vi "Vehicle.vi"(8 "error in (no error)":errorcluster, 9 "Logger In":refnum<queue>, 10 "Pipeline In":refnum<queue>, 11 "Vehicle Queue In":refnum<queue>) -> (0 "error out":errorcluster, 3 "Vehicle Queue Out":refnum<queue>)   [LabVIEW 2016]
uses:
  Message Format.ctl
  StateDef_generic.ctl
  StateData_Vehicle.ctl
  <vilib>/addons/zeromq/socket_type.ctl
  <vilib>/addons/zeromq/socket_options.ctl
  <vilib>/addons/zeromq/zmq_socket.lvclass
  <vilib>/addons/zeromq/zmq_context.lvclass
  <vilib>/addons/zeromq/zeromq.lvlib
panel:
  out "Vehicle  Sensors":cluster{dbl, dbl, dbl}(graph)
  # "VEHICLE DATA"
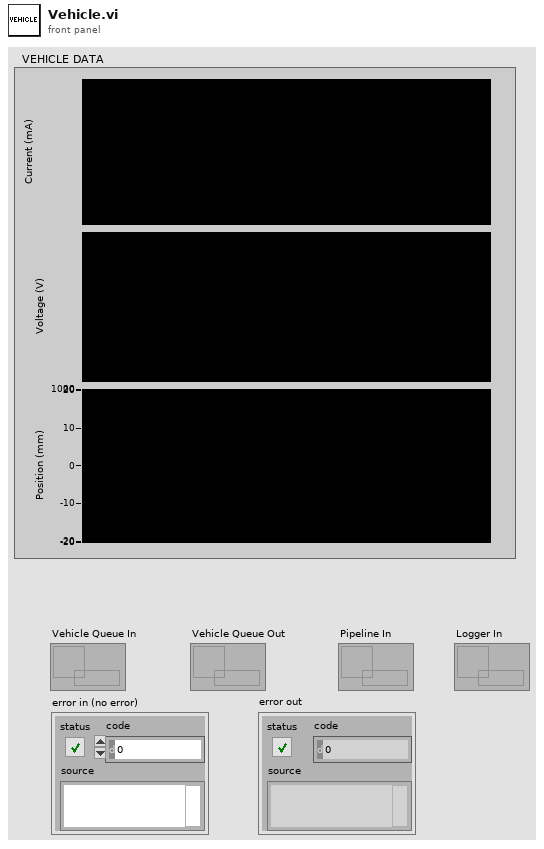
[diagram p1: front panel]
types:
  T1 = typedef "StateData_Vehicle.ctl" = cluster{"Current":dbl, "Voltage":dbl, "Position":dbl}
  T2 = typedef "StateDef_generic.ctl" = enum16{"Initialize", "Running", "Exit"}
  T3 = typedef "zeromq.lvlib/socket_options.ctl" = enum8{"NONE", "ZMQ_HWM", "<2>", "ZMQ_SWAP", "ZMQ_AFFINITY", "ZMQ_IDENTITY", "ZMQ_SUBSCRIBE", "ZMQ_UNSUBSCRIBE", "ZMQ_RATE", "ZMQ_RECOVERY_IVL", "ZMQ_MCAST_LOOP", "ZMQ_SNDBUF", "ZMQ_RCVBUF", "ZMQ_RCVMORE", "ZMQ_FD", "ZMQ_EVENTS", "ZMQ_TYPE", "ZMQ_LINGER", "ZMQ_RECONNECT_IVL", "ZMQ_BACKLOG", "ZMQ_RECOVERY_IVL_MSEC", "ZMQ_RECONNECT_IVL_MAX", "ZMQ_MAXMSGSIZE", "ZMQ_SNDHWM", "ZMQ_RCVHWM", "ZMQ_MULTICAST_HOPS", "<26>", "ZMQ_RCVTIMEO", "ZMQ_SNDTIMEO", "<29>", "<30>", "ZMQ_IPV4ONLY", "ZMQ_LAST_ENDPOINT", "ZMQ_ROUTER_MANDATORY", "ZMQ_TCP_KEEPALIVE", "ZMQ_TCP_KEEPALIVE_CNT", "ZMQ_TCP_KEEPALIVE_IDLE", "ZMQ_TCP_KEEPALIVE_INTVL", "ZMQ_TCP_ACCEPT_FILTER", "ZMQ_DELAY_ATTACH_ON_CONNECT", "ZMQ_XPUB_VERBOSE"}
  T4 = typedef "zeromq.lvlib/socket_type.ctl" = enum8{"ZMQ_PAIR", "ZMQ_PUB", "ZMQ_SUB", "ZMQ_REQ", "ZMQ_REP", "ZMQ_DEALER", "ZMQ_ROUTER", "ZMQ_PULL", "ZMQ_PUSH", "ZMQ_XPUB", "ZMQ_XSUB"}
  T5 = typedef "Message Format.ctl" = cluster{"header":string, "data":variant}
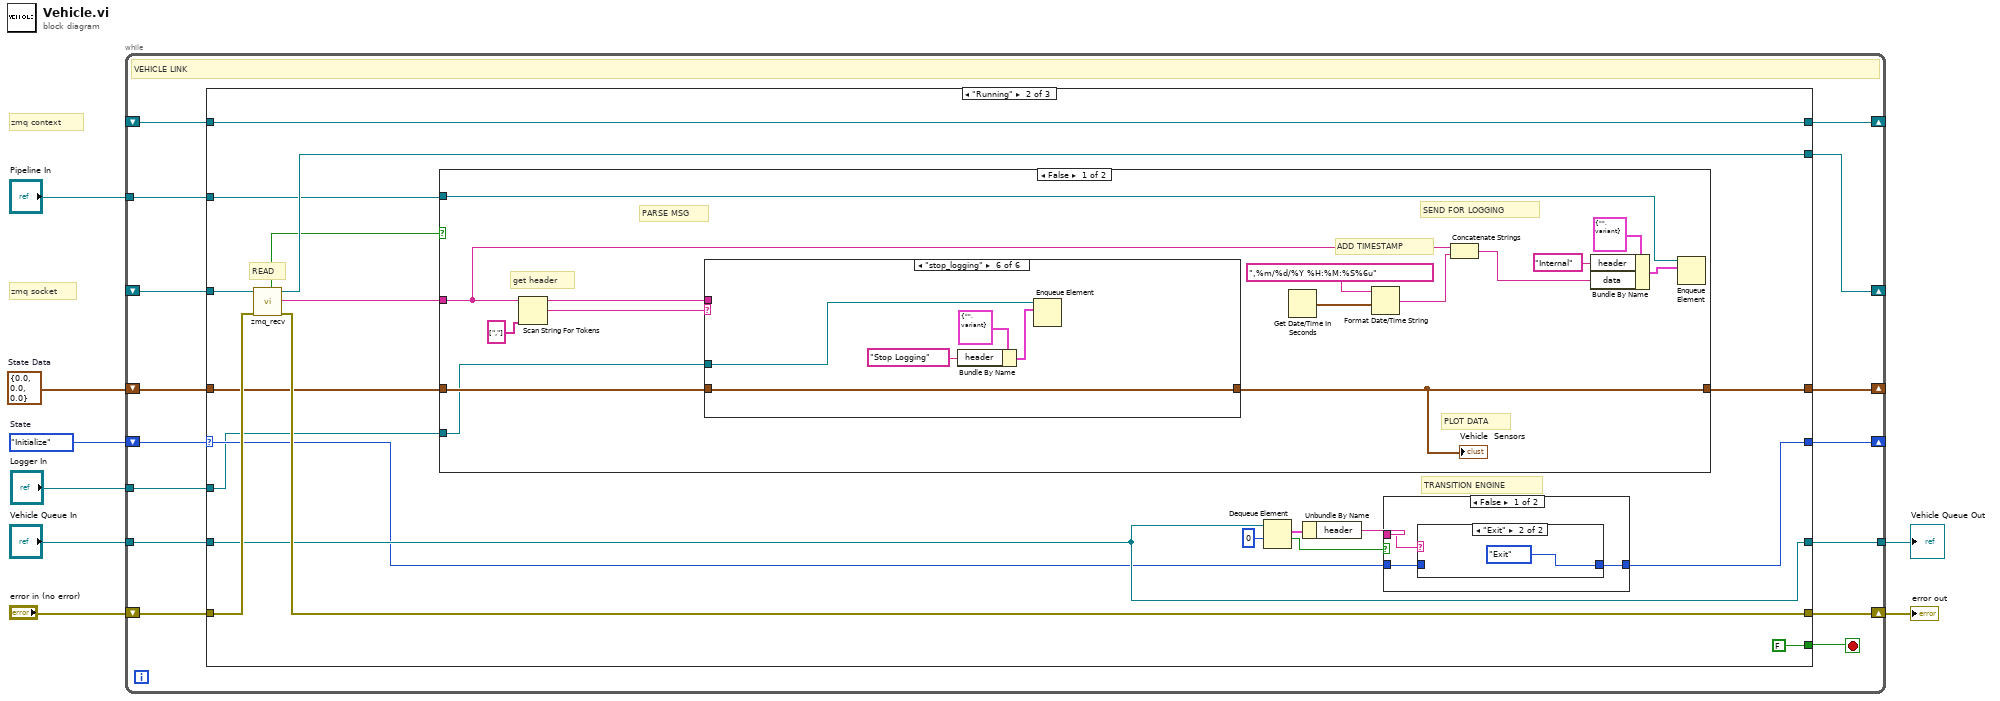
[diagram p0: block diagram]
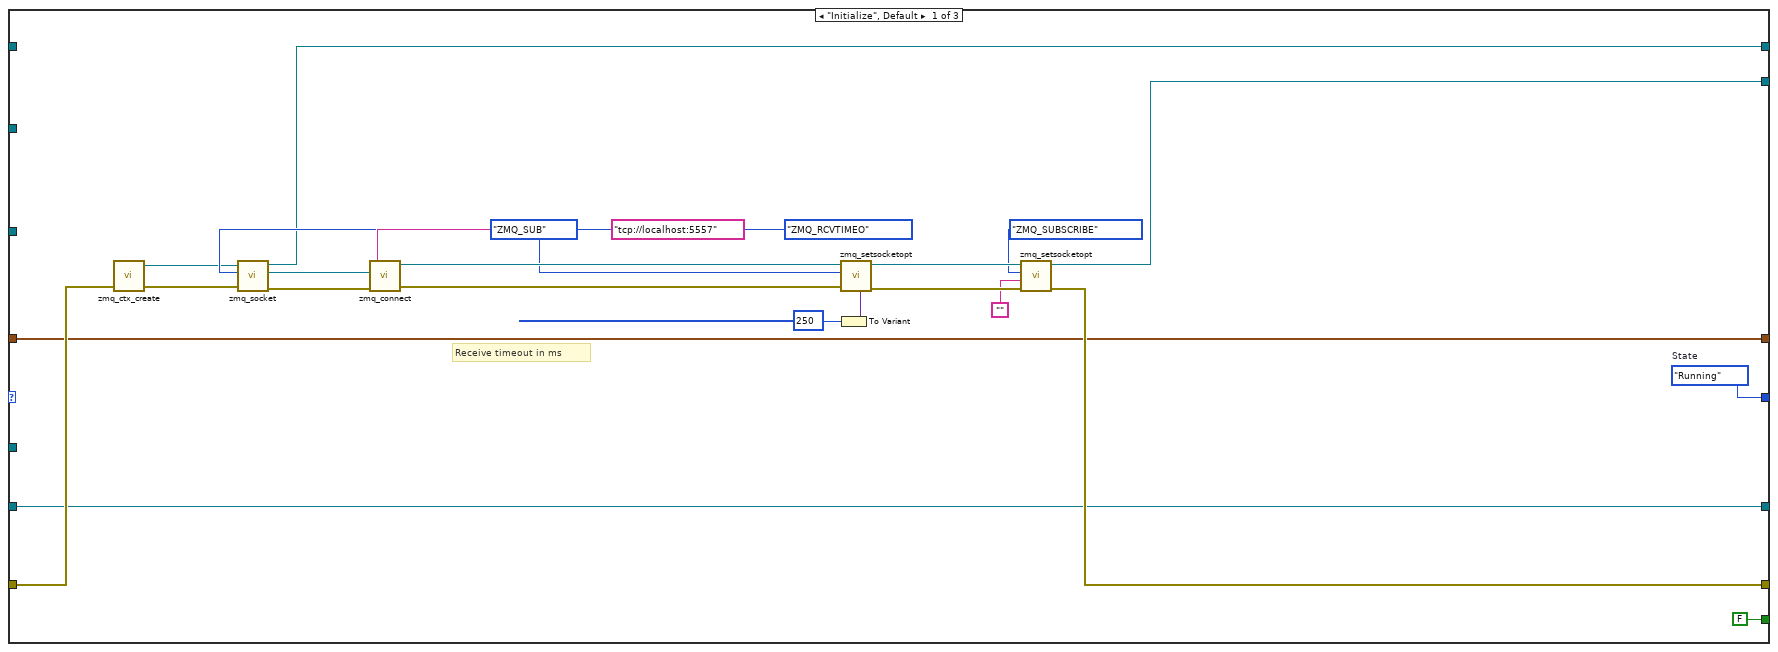
[diagram p2: hidden frame]
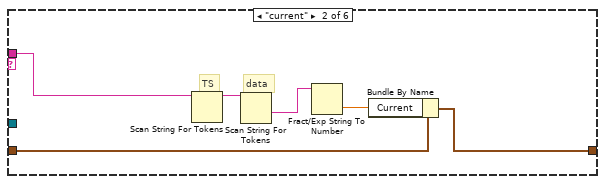
[diagram p6: hidden frame]
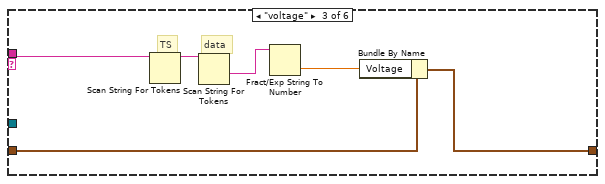
[diagram p7: hidden frame]
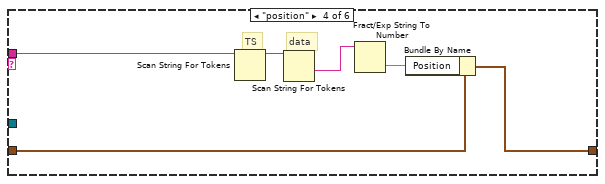
[diagram p8: hidden frame]
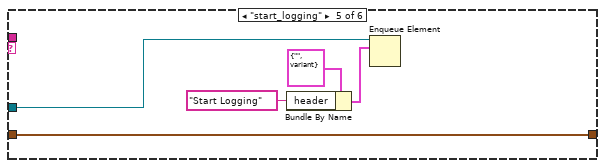
[diagram p9: hidden frame]
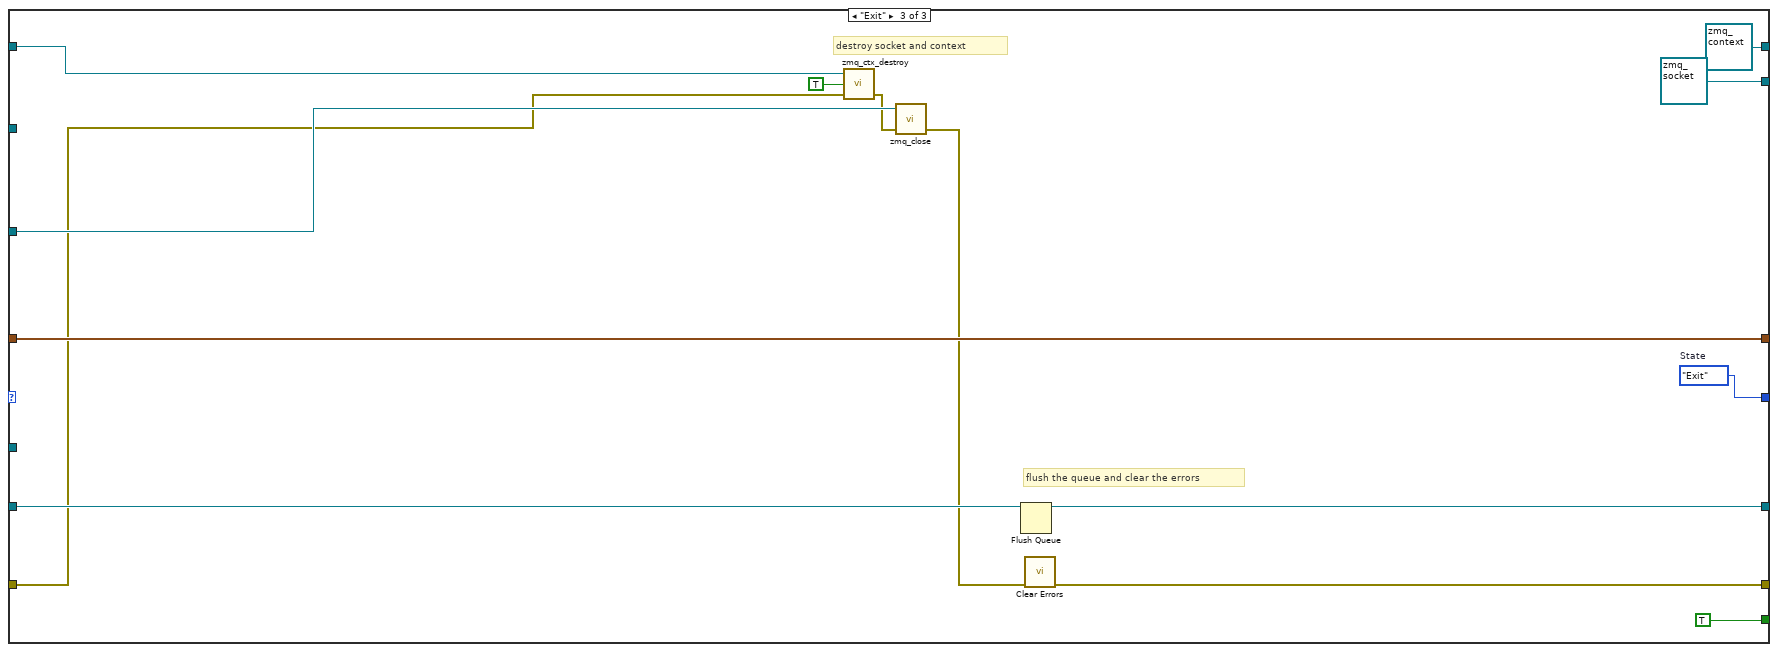
[diagram p11: hidden frame]
diagram:
  w3 = T1 {"Current"=0.0, "Voltage"=0.0, "Position"=0.0}  # State Data
  w5 = StateDef_generic."Initialize"  # State
  # "zmq socket"
  # "zmq context"
  n1 = while {
    shift-right: [w23] -> w4
    shift-left: "error in (no error)" -> [w17]
    shift-right: [w22] -> _
    shift-left: _ -> [w21]
    shift-right: [w20] -> _
    shift-left: _ -> [w19]
    tunnel: "Pipeline In" -> [w15]
    tunnel: "Vehicle Queue In" -> [w16]
    shift-right: [w13] -> _
    shift-left: w5 -> [w18]
    shift-right: [w11] -> _
    shift-left: w3 -> [w12]
    tunnel: [w10] -> w2
    tunnel: "Logger In" -> [w9]
    stop <- w14 stop-if-true
    # "VEHICLE LINK"
    n2 = case shown="\"Running\"" w18 {
      selector: w18 -> [_ w49 _]
      tunnel: [w28 w63 w120] -> w23
      tunnel: [w33 w62 refnum<class "zmq_socket.lvclass"> refnum ("socket out")] -> w22
      tunnel: w21 -> [_ w64 w129]
      tunnel: [w32 w65 refnum<class "zmq_context.lvclass"> refnum ("context out")] -> w20
      tunnel: w19 -> [_ w65 w130]
      tunnel: w17 -> [w29 w60 w119]
      tunnel: w16 -> [w24 w51 w124]
      tunnel: w15 -> [_ w56 _]
      tunnel: [FALSE FALSE TRUE] -> w14
      tunnel: [w26 w48 w126] -> w13
      tunnel: w12 -> [w25 w57 w125]
      tunnel: [w25 w55 w125] -> w11
      tunnel: [w24 w51 w118] -> w10
      tunnel: w9 -> [_ w47 _]
      frame "Initialize", Default {
        w26 = StateDef_generic."Running"  # State
        # "Receive timeout in ms"
        n3 = call <vilib>:"zmq_ctx_create.vi"("error in"=w29) -> ("error out"=w39:errorcluster, "context out"=w38:refnum<class "zmq_context.lvclass">)  [unwired: 3 in]
        n4 = call <vilib>:"zmq_socket.vi"("error in"=w39, "socket type"=socket_type."ZMQ_SUB", "context in"=w38) -> ("error out"=w42:errorcluster, "socket out"=w41:refnum<class "zmq_socket.lvclass">, "context out"=w32:refnum<class "zmq_context.lvclass">)  [unwired: 2 in]
        n5 = call <vilib>:"zmq_connect.vi"("error in"=w42, "endpoint"="tcp://localhost:5557", "socket in"=w41) -> ("error out"=w46:errorcluster, "socket out"=w45:refnum<class "zmq_socket.lvclass">)  [unwired: 1 in]
        n6 = To Variant(anything=250) -> (Variant=w30:variant)
        n7 = call <vilib>:"zmq_setsocketopt.vi"("error in"=w46, "value"=w30, "option"=socket_options."ZMQ_RCVTIMEO", "socket in"=w45) -> ("error out"=w36:errorcluster, "socket out"=w37:refnum<class "zmq_socket.lvclass">)  [unwired: 2 in]
        n8 = call <vilib>:"zmq_setsocketopt.vi"("error in"=w36, "value"="", "option"=socket_options."ZMQ_SUBSCRIBE", "socket in"=w37) -> ("error out"=w28:errorcluster, "socket out"=w33:refnum<class "zmq_socket.lvclass">)  [unwired: 2 in]
      }
      frame "Running" {
        # "TRANSITION ENGINE"
        # "READ"
        n9 = call <vilib>:"zmq_recv.vi"("error in"=w60, "socket in"=w64) -> ("error out"=w63:errorcluster, "data"=w58:string, "socket out"=w62:refnum<class "zmq_socket.lvclass">, "timeout?"=w61:bool)  [unwired: 3 in, 1 out]
        n10 = case shown="False" w61 {
          tunnel: w58 -> [w79 _]
          tunnel: w57 -> [w77 w116]
          tunnel: [w76 w116] -> w55
          tunnel: w56 -> [w75 _]
          tunnel: w47 -> [w72 _]
          frame False {
            # "ADD TIMESTAMP"
            # "SEND FOR LOGGING"
            # "PLOT DATA"
            # "PARSE MSG"
            # "get header"
            n11 = Scan String For Tokens(6:string[] [","], 9:w79) -> (1:w74:string, 3:w73:string)  [unwired: 4 in, 2 out]
            n12 = case shown="\"stop_logging\"" w74 {
              tunnel: [w87 w92 w98 w104 w110 w115] -> w76
              tunnel: w77 -> [w87 w93 w99 w105 w110 w115]
              tunnel: w73 -> [_ w89 w94 w101 _ _]
              tunnel: w72 -> [_ _ _ _ w109 w114]
              frame "other", Default {
              }
              frame "current" {
                # "data"
                # "TS"
                n13 = Scan String For Tokens(9:w89) -> (3:w91:string)  [unwired: 5 in, 3 out]
                n14 = Scan String For Tokens(9:w91) -> (1:w90:string)  [unwired: 5 in, 3 out]
                n15 = Fract/Exp String To Number(string=w90) -> (number=w88:dbl)  [unwired: 3 in, 1 out]
                n16 = Bundle By Name(cluster=w93, "Current"=w88) -> (w92:T1)
              }
              frame "voltage" {
                # "data"
                # "TS"
                n17 = Scan String For Tokens(9:w94) -> (3:w97:string)  [unwired: 5 in, 3 out]
                n18 = Scan String For Tokens(9:w97) -> (1:w96:string)  [unwired: 5 in, 3 out]
                n19 = Fract/Exp String To Number(string=w96) -> (number=w95:dbl)  [unwired: 3 in, 1 out]
                n20 = Bundle By Name(cluster=w99, "Voltage"=w95) -> (w98:T1)
              }
              frame "position" {
                # "data"
                # "TS"
                n21 = Scan String For Tokens(9:w101) -> (3:w103:string)  [unwired: 5 in, 3 out]
                n22 = Scan String For Tokens(9:w103) -> (1:w102:string)  [unwired: 5 in, 3 out]
                n23 = Fract/Exp String To Number(string=w102) -> (number=w100:dbl)  [unwired: 3 in, 1 out]
                n24 = Bundle By Name(cluster=w105, "Position"=w100) -> (w104:T1)
              }
              frame "start_logging" {
                n25 = Bundle By Name(cluster=T5 {"header"="", "data"=variant} ("msg format"), "header"="Start Logging") -> (w106:T5)
                n26 = Enqueue Element(queue=w109, element=w106) -> ()  [unwired: 2 in, 3 out]
              }
              frame "stop_logging" {
                n27 = Bundle By Name(cluster=T5 {"header"="", "data"=variant} ("msg format"), "header"="Stop Logging") -> (w111:T5)
                n28 = Enqueue Element(queue=w114, element=w111) -> ()  [unwired: 2 in, 3 out]
              }
            }
            "Vehicle  Sensors" <- w76
            n29 = Get Date/Time In Seconds() -> (seconds since 1Jan1904=w82:timestamp)
            n30 = Format Date/Time String(time format string (%c)=",%m/%d/%Y %H:%M:%S%6u", seconds (now)=w82) -> (date/time string=w80:string)  [unwired: 1 in]
            n31 = Concatenate Strings(w79, w80) -> (w78:string)
            n32 = Bundle By Name(cluster=T5 {"header"="", "data"=variant} ("msg format"), "header"="Internal", "data"=w78) -> (w83:T5)
            n33 = Enqueue Element(queue=w75, element=w83) -> ()  [unwired: 2 in, 3 out]
          }
          frame True {
          }
        }
        n34 = Dequeue Element(queue=w51, timeout in ms (-1)=0) -> (element=w53:T5, timed out?=w50:bool)  [unwired: 1 in, 2 out]
        n35 = Unbundle By Name(w53) -> ("header"=w52:string)
        n36 = case shown="False" w50 {
          tunnel: w52 -> [w68 _]
          tunnel: [w67 w71] -> w48
          tunnel: w49 -> [w66 w71]
          frame False {
            n37 = case shown="\"Exit\"" w68 {
              tunnel: [w69 StateDef_generic."Exit" ("State")] -> w67
              tunnel: w66 -> [w69 _]
              frame "any other", Default {
              }
              frame "Exit" {
              }
            }
          }
          frame True {
          }
        }
      }
      frame "Exit" {
        w126 = StateDef_generic."Exit"  # State
        # "destroy socket and context"
        # "flush the queue and clear the errors"
        n38 = call <vilib>:"zmq_ctx_destroy.vi"("error in"=w119, "reap? (F)"=TRUE, "context in"=w130) -> ("error out"=w121:errorcluster)  [unwired: 2 in]
        n39 = call <vilib>:"zmq_close.vi"("error in"=w121, "socket"=w129) -> ("error out"=w117:errorcluster)  [unwired: 3 in]
        n40 = Flush Queue(queue=w124) -> (queue out=w118:refnum<queue>)  [unwired: 1 in, 2 out]
        n41 = call <vilib>:"Clear Errors.vi"("error in (no error)"=w117) -> ("error out"=w120:errorcluster)  [unwired: 5 in, 1 out]
      }
    }
  }
  "error out" <- w4
  "Vehicle Queue Out" <- w2
